vi "Run.vi"(7 "Team Index":i32, 8 "Column":i32, 9 "Row":i32, 10 "View":i32[](array[numeric]) caption="View (Team Index, -1: empty)", 11 "64 In":refnum<class "Border.lvclass">) -> (0 "Replicated":refnum<class "Square.lvclass">, 1 "Direction":T1, 2 "Action":T2, 3 "64 Out":refnum<class "Border.lvclass">)   [LabVIEW 2015, in "Border.lvclass"]
uses:
  Border.lvclass
  Type Defs/Action Enum.ctl
  Type Defs/Direction Enum.ctl
  Square/Square.lvclass
  Border.lvclass/Border.ctl
  Border Type.ctl
  Assassin/Assassin.lvclass
  SubVIs/Read-Only Globals.vi
  Common/Find Enemy.vi
  SubVIs/Globals (private).vi
  Common/Common.lvlib
  Type Defs/SB Type Defs.lvlib
panel:
  # "NW\nN\nNE\nE\nSE\nS\nSW\nW"
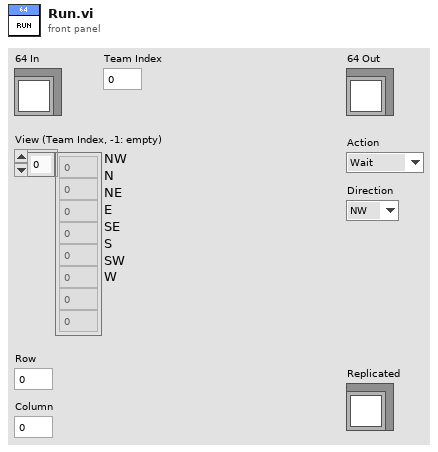
[diagram p1: front panel]
types:
  T1 = typedef "SB Type Defs.lvlib/Direction Enum.ctl" = enum16{"NW", "N", "NE", "E", "SE", "S", "SW", "W"}
  T2 = typedef "SB Type Defs.lvlib/Action Enum.ctl" = enum16{"Wait", "Move", "Attack", "Replicate"}
  T3 = typedef "Border.lvclass/Border Type.ctl" = enum16{"Starter", "Assassin", "Line Starter", "ELine", "WLine", "StartPatrol", "Patrol", "Wall"}
  T4 = typedef "Common.lvlib/Position.ctl" = cluster{"Column":i32, "Row":i32}
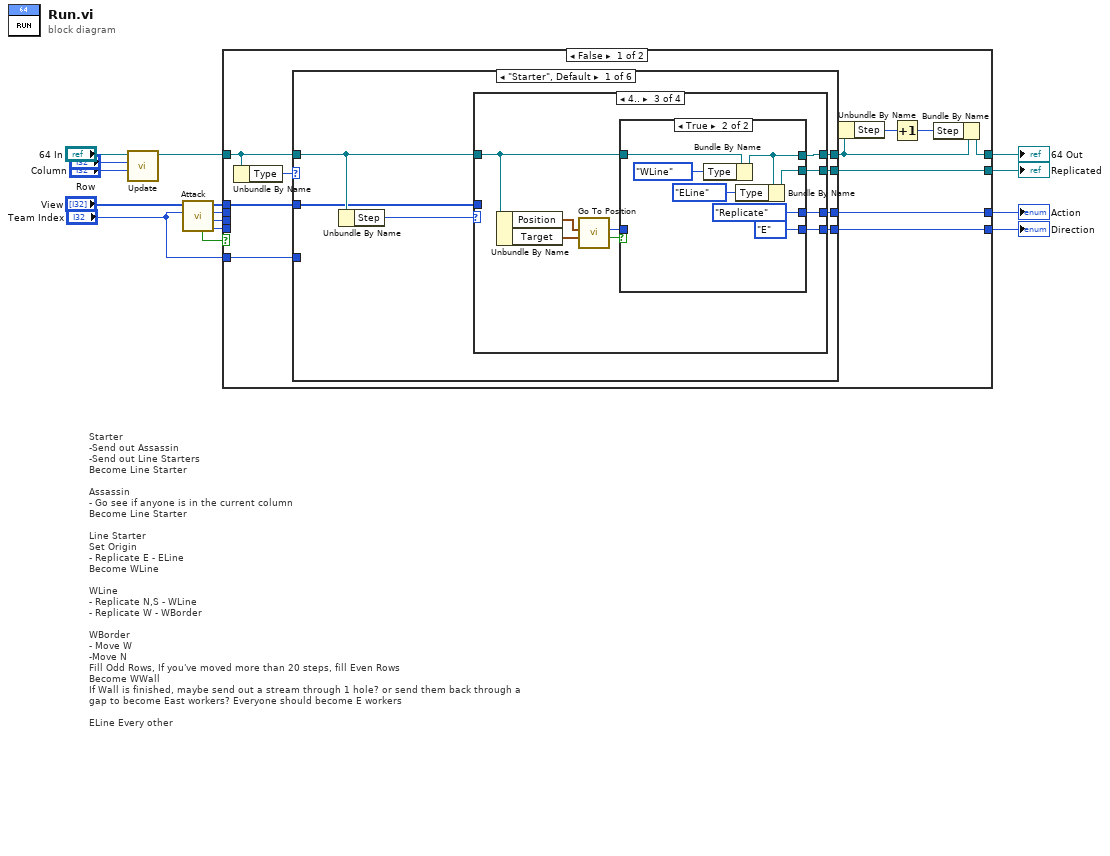
[diagram p0: block diagram]
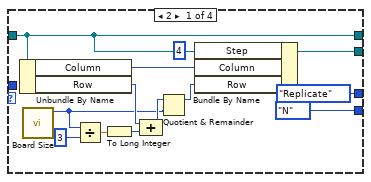
[diagram p2: hidden frame]
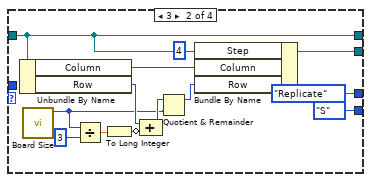
[diagram p3: hidden frame]
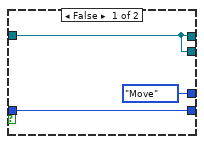
[diagram p4: hidden frame]
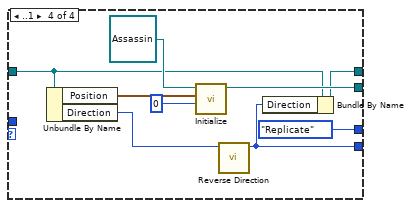
[diagram p5: hidden frame]
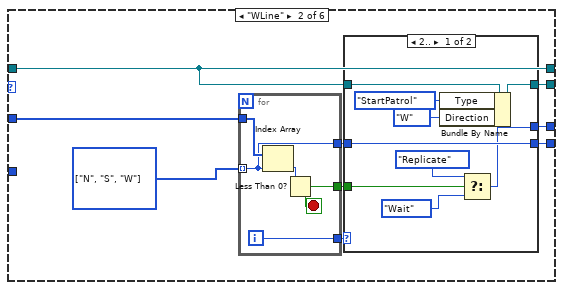
[diagram p6: hidden frame]
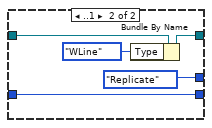
[diagram p7: hidden frame]
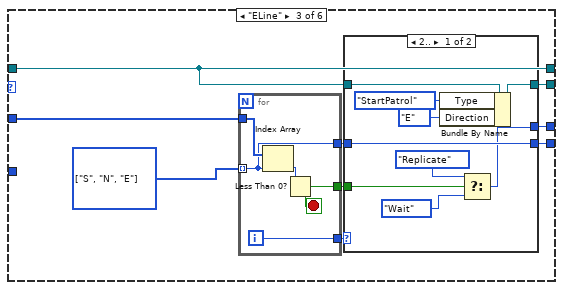
[diagram p8: hidden frame]
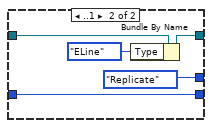
[diagram p9: hidden frame]
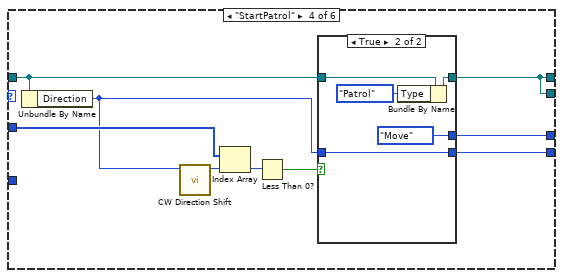
[diagram p10: hidden frame]
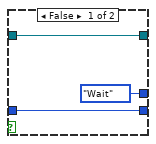
[diagram p11: hidden frame]
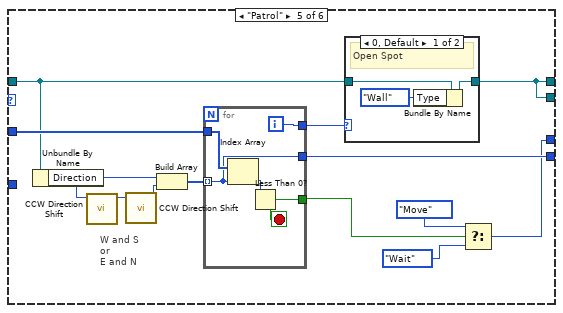
[diagram p12: hidden frame]
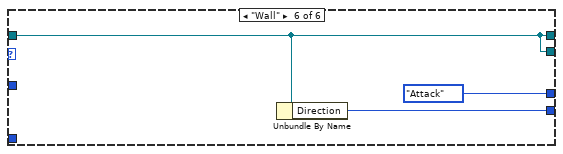
[diagram p14: hidden frame]
diagram:
  # "Starter\n-Send out Assassin\n-Send out Line Starters\nBecome Line Starter\n\nAssassin\n- Go see if anyone is in the current column\nBecome Line Starter\n\nLine Starter\nSet Origin\n- Replicate E - ELine\nBecome WLine\n\nWLine\n- Replicate N,S - WLine\n- Replicate W - WBorder\n\nWBorder\n- Move W\n-Move N\nFill Odd Rows, If you've moved more than 20 steps, fill Even Rows\nBecome WWall\nIf Wall is finished, maybe send out a stream through 1 hole? or send them back through a gap to become East workers? Everyone should become E workers\n\nELine Every other"
  n1 = call "Update.vi"("Column"="Column", "Row"="Row", "64 in"="64 In") -> ("64 out"=w9:refnum<class "Border.lvclass">)  [unwired: 8 in]
  n2 = call "Attack.vi"("Team Index"="Team Index", "View"="View") -> ("Enemy"=w2:i32, "Direction"=w3:i32, "Action"=w4:T2, "View"=w5:i32[], "Enemy Found?"=w7:bool)  [unwired: 4 in, 1 out]
  n3 = case shown="False" w7 {
    tunnel: [w26 w186] -> w12
    tunnel: [w18 w186] -> w1
    tunnel: [w25 w188] -> w11
    tunnel: [w24 w187] -> w10
    tunnel: w5 -> [w23 _]
    tunnel: "Team Index" -> [w22 _]
    tunnel: w9 -> [w21 w186]
    tunnel: w4 -> [_ w188]
    tunnel: w3 -> [_ w187]
    tunnel: w2 -> [_ _]
    frame False {
      n4 = Unbundle By Name(w21) -> ("Type"=w20:T3)
      n5 = case shown="\"Starter\", Default" w20 {
        tunnel: w21 -> [w29 w90 w118 w146 w165 w184]
        tunnel: [w33 w89 w117 w150 w170 w184] -> w26
        tunnel: [w31 w90 w118 w150 w170 w184] -> w19
        tunnel: [w32 w95 w123 w152 w166 Action_Enum."Attack" ("Action")] -> w25
        tunnel: [w30 w93 w121 w151 w172 w183] -> w24
        tunnel: w23 -> [w27 w92 w120 w149 w173 _]
        tunnel: w22 -> [_ _ _ _ _ _]
        frame "Starter", Default {
          n6 = Unbundle By Name(w29) -> ("Step"=w28:i32)
          n7 = case shown="4.." w28 {
            tunnel: [w44 w57 w60 w86] -> w33
            tunnel: w29 -> [w43 w56 w66 w85]
            tunnel: [Action_Enum."Replicate" ("Action") Action_Enum."Replicate" ("Action") w65 Action_Enum."Replicate" ("Action")] -> w32
            tunnel: [w43 w56 w61 w81] -> w31
            tunnel: [Direction_Enum."N" ("Direction") Direction_Enum."S" ("Direction") w63 w80] -> w30
            tunnel: w27 -> [_ _ _ _]
            frame 2 {
              n8 = Unbundle By Name(w43) -> ("Column"=w42:i32, "Row"=w41:i32)
              n9 = call "Board Size.vi"() -> ("Board Size"=w35:i32)  [unwired: 11 in]
              n10 = Divide(x=w35, y=3) -> (x/y=w39:dbl)
              n11 = To Long Integer(number=w39) -> (32bit integer=w38:i32)
              n12 = Compound Arithmetic op=ADD(w41, w38) -> (w36:i32)
              n13 = Quotient & Remainder(x=w36, y=w35) -> (x-y*floor(x/y)=w37:i32)  [unwired: 1 out]
              n14 = Bundle By Name(cluster=w43, "Step"=4, "Column"=w42, "Row"=w37) -> (w44:refnum<class "Border.lvclass">)
            }
            frame 3 {
              n15 = Unbundle By Name(w56) -> ("Column"=w55:i32, "Row"=w54:i32)
              n16 = call "Board Size.vi"() -> ("Board Size"=w48:i32)  [unwired: 11 in]
              n17 = Divide(x=w48, y=3) -> (x/y=w52:dbl)
              n18 = To Long Integer(number=w52) -> (32bit integer=w51:i32)
              n19 = Compound Arithmetic op=ADD(w54, invert w51) -> (w49:i32)
              n20 = Quotient & Remainder(x=w49, y=w48) -> (x-y*floor(x/y)=w50:i32)  [unwired: 1 out]
              n21 = Bundle By Name(cluster=w56, "Step"=4, "Column"=w55, "Row"=w50) -> (w57:refnum<class "Border.lvclass">)
            }
            frame 4.. {
              n22 = Unbundle By Name(w66) -> ("Position"=w68:T4, "Target"=w67:T4)
              n23 = call "Go To Position.vi"("Target Position"=w67, "My Position"=w68) -> ("Arrived?"=w62:bool, "Direction"=w64:T1)  [unwired: 7 in, 1 out]
              n24 = case shown="True" w62 {
                tunnel: w66 -> [w71 w78]
                tunnel: [w71 w74] -> w61
                tunnel: [Action_Enum."Move" ("Action") Action_Enum."Replicate" ("Action")] -> w65
                tunnel: w64 -> [w70 _]
                tunnel: [w70 Direction_Enum."E" ("Direction")] -> w63
                tunnel: [w71 w73] -> w60
                frame False {
                }
                frame True {
                  n25 = Bundle By Name(cluster=w78, "Type"=Border_Type."WLine") -> (w74:refnum<class "Border.lvclass">)
                  n26 = Bundle By Name(cluster=w74, "Type"=Border_Type."ELine") -> (w73:refnum<class "Border.lvclass">)
                }
              }
            }
            frame ..1 {
              n27 = Unbundle By Name(w85) -> ("Position"=w84:T4, "Direction"=w82:T1)
              n28 = call "Initialize.vi"("Current Target"=0, "Position"=w84, "Assassin in"=refnum<class "Assassin.lvclass"> refnum ("Assassin.lvclass")) -> ("Assassin out"=w86:refnum<class "Assassin.lvclass">)  [unwired: 8 in]
              n29 = call "Reverse Direction.vi"("Direction in"=w82) -> ("Reverse Direction"=w80:i32)  [unwired: 10 in]
              n30 = Bundle By Name(cluster=w85, "Direction"=w80) -> (w81:refnum<class "Border.lvclass">)
            }
          }
        }
        frame "WLine" {
          w96 = T1[] [enum."N", enum."S", enum."W"] items=["NW", "N", "NE", "E", "SE", "S", "SW", "W"]
          n31 = for {
            tunnel: w92 -> [w115]
            tunnel: w96 -> [w112] mode=indexing
            tunnel: [w113] -> w88
            tunnel: [w112] -> w94
            tunnel: [w111] -> w91
            i -> [w111]
            stop <- w113 stop-if-true
            n32 = Index Array(array=w115, index=w112) -> (element=w114:i32)
            n33 = Less Than 0?(x=w114) -> (x < 0?=w113:bool)
          }
          n34 = case shown="2.." w91 {
            tunnel: [w100 Action_Enum."Replicate" ("t")] -> w95
            tunnel: w94 -> [w103 w109]
            tunnel: [w103 w109] -> w93
            tunnel: w90 -> [w105 w108]
            tunnel: [w99 w107] -> w89
            tunnel: w88 -> [w104 _]
            frame 2.. {
              n35 = Bundle By Name(cluster=w105, "Type"=Border_Type."StartPatrol", "Direction"=Direction_Enum."W") -> (w99:refnum<class "Border.lvclass">)
              n36 = Select(t=Action_Enum."Replicate" ("Action"), s=w104, f=Action_Enum."Wait" ("Action")) -> (s? t:f=w100:T2)
            }
            frame ..1 {
              n37 = Bundle By Name(cluster=w108, "Type"=Border_Type."WLine") -> (w107:refnum<class "Border.lvclass">)
            }
          }
        }
        frame "ELine" {
          w124 = T1[] [enum."S", enum."N", enum."E"] items=["NW", "N", "NE", "E", "SE", "S", "SW", "W"]
          n38 = for {
            tunnel: w120 -> [w143]
            tunnel: w124 -> [w140] mode=indexing
            tunnel: [w141] -> w116
            tunnel: [w140] -> w122
            tunnel: [w139] -> w119
            i -> [w139]
            stop <- w141 stop-if-true
            n39 = Index Array(array=w143, index=w140) -> (element=w142:i32)
            n40 = Less Than 0?(x=w142) -> (x < 0?=w141:bool)
          }
          n41 = case shown="2.." w119 {
            tunnel: [w128 Action_Enum."Replicate" ("t")] -> w123
            tunnel: w122 -> [w131 w137]
            tunnel: [w131 w137] -> w121
            tunnel: w118 -> [w133 w136]
            tunnel: [w127 w135] -> w117
            tunnel: w116 -> [w132 _]
            frame 2.. {
              n42 = Bundle By Name(cluster=w133, "Type"=Border_Type."StartPatrol", "Direction"=Direction_Enum."E") -> (w127:refnum<class "Border.lvclass">)
              n43 = Select(t=Action_Enum."Replicate" ("Action"), s=w132, f=Action_Enum."Wait" ("Action")) -> (s? t:f=w128:T2)
            }
            frame ..1 {
              n44 = Bundle By Name(cluster=w136, "Type"=Border_Type."ELine") -> (w135:refnum<class "Border.lvclass">)
            }
          }
        }
        frame "StartPatrol" {
          n45 = Unbundle By Name(w146) -> ("Direction"=w145:T1)
          n46 = call "CW Direction Shift.vi"("Direction"=w145) -> ("Numeric"=w144:i32)  [unwired: 10 in]
          n47 = Index Array(array=w149, index=w144) -> (element=w148:i32)
          n48 = Less Than 0?(x=w148) -> (x < 0?=w147:bool)
          n49 = case shown="True" w147 {
            tunnel: [Action_Enum."Wait" ("Action") Action_Enum."Move" ("Action")] -> w152
            tunnel: [w153 w156] -> w151
            tunnel: [w155 w159] -> w150
            tunnel: w146 -> [w155 w157]
            tunnel: w145 -> [w153 w156]
            frame False {
            }
            frame True {
              n50 = Bundle By Name(cluster=w157, "Type"=Border_Type."Patrol") -> (w159:refnum<class "Border.lvclass">)
            }
          }
        }
        frame "Patrol" {
          # "W and S\nor\nE and N"
          n51 = Unbundle By Name(w165) -> ("Direction"=w163:T1)
          n52 = call "CCW Direction Shift.vi"("Direction"=w163) -> ("Numeric"=w164:i32)  [unwired: 10 in]
          n53 = call "CCW Direction Shift.vi"("Direction"=w164) -> ("Numeric"=w162:i32)  [unwired: 10 in]
          n54 = Build Array(w163, w162) -> (w161:i32[])
          n55 = for {
            tunnel: w173 -> [w182]
            tunnel: w161 -> [w179] mode=indexing
            tunnel: [w180] -> w167
            tunnel: [w179] -> w172
            tunnel: [w178] -> w171
            i -> [w178]
            stop <- w180 stop-if-true
            n56 = Index Array(array=w182, index=w179) -> (element=w181:i32)
            n57 = Less Than 0?(x=w181) -> (x < 0?=w180:bool)
          }
          n58 = case shown="0, Default" w171 {
            tunnel: w165 -> [w176 w177]
            tunnel: [w175 w177] -> w170
            frame 0, Default {
              # "Open Spot"
              n59 = Bundle By Name(cluster=w176, "Type"=Border_Type."Wall") -> (w175:refnum<class "Border.lvclass">)
            }
            frame 1 {
              # "Patrol"
            }
          }
          n60 = Select(t=Action_Enum."Move" ("Action"), s=w167, f=Action_Enum."Wait" ("Action")) -> (s? t:f=w166:T2)
        }
        frame "Wall" {
          n61 = Unbundle By Name(w184) -> ("Direction"=w183:T1)
        }
      }
      n62 = Unbundle By Name(w19) -> ("Step"=w17:i32)
      n63 = Increment(x=w17) -> (x+1=w16:i32)
      n64 = Bundle By Name(cluster=w19, "Step"=w16) -> (w18:refnum<class "Border.lvclass">)
    }
    frame True {
    }
  }
  "64 Out" <- w1
  "Action" <- w11
  "Direction" <- w10
  "Replicated" <- w12
